vi "Fluence in multiple areas.vi"(0 "Analyze Fluence in":refnum<class "Analyze Fluence.lvclass">, 5 "Image in":T2, 7 "Energy":dbl[unit], 11 "error in (no error)":errorcluster) -> (4 "Analyze Fluence out":refnum<class "Analyze Fluence.lvclass">, 6 "Image Dst Out":T2, 8 "Max Fluence J/cm^2":dbl[unit], 10 "fluence infos":T3[](array[typedef]), 15 "error out":errorcluster)   [LabVIEW 2014, in "Analyze.lvlib" / "Analyze Fluence.lvclass"]
uses:
  Analyze Fluence.lvclass
  Fluence Info.ctl
  <vilib>/vision/Image Controls.llb/IMAQ Image.ctl
  Analyze Parameter/Analyze Parameter Fluence/Analyze Parameter Fluence.lvclass
  Analyze Fluence.lvclass/Analyze Fluence.ctl
  <vilib>/vision/NI_Vision_Development_Module.lvlib
  Analyze BaseClass/Analyze BaseClass/Analyze BaseClass.lvclass
panel:
  in  "ROI Descriptor out":T1 {"Contours"."Type" items=["No Selection", "Point", "Line", "Rectangle", "Oval", "Polygon", "Freehand Region", "Annulus", "Unused2", "Unused3", "Broken Line", "Freehand Line", "Rotated Rectangle"]}
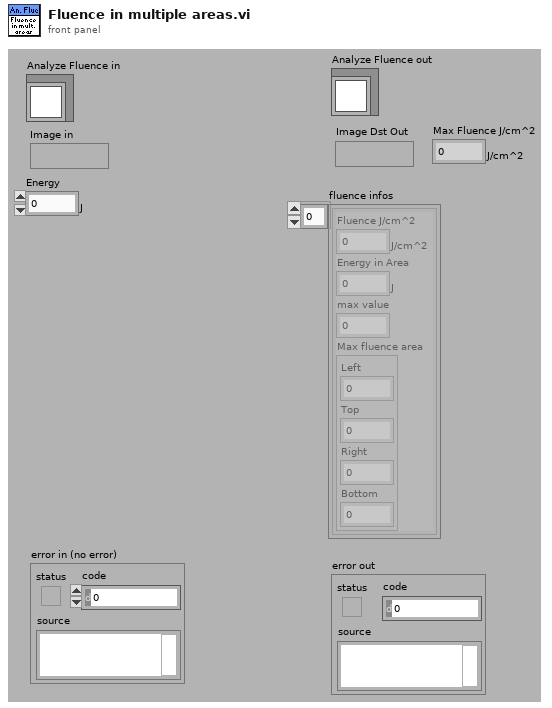
[diagram p1: front panel]
types:
  T1 = typedef "ROI Descriptor" = cluster{"Global Rectangle":i32[], "Contours":cluster{"ID":enum32{"External", "Internal"}, "Type":u32, "Coordinates":i32[]}[]}
  T2 = typedef "IMAQ Image.ctl" = refnum<image>
  T3 = typedef "Analyze.lvlib/Analyze Fluence.lvclass/Fluence Info.ctl" = cluster{"Fluence J/cm^2":dbl[unit], "Energy in Area":dbl[unit], "max value":i64, "Max fluence area":cluster{"Left":i32, "Top":i32, "Right":i32, "Bottom":i32}}
  T4 = typedef "Image Type" = u32
  T5 = typedef "IMAQ Rectangle" = cluster{"Left":i32, "Top":i32, "Right":i32, "Bottom":i32, "Rotation":dbl}
  T6 = cluster{"Left":i32, "Top":i32, "Right":i32, "Bottom":i32}
  T7 = cluster{"Fluence J/cm^2":dbl[unit], "Energy in Area":dbl[unit], "max value":i64, "Max fluence area":cluster{"Left":i32, "Top":i32, "Right":i32, "Bottom":i32}}
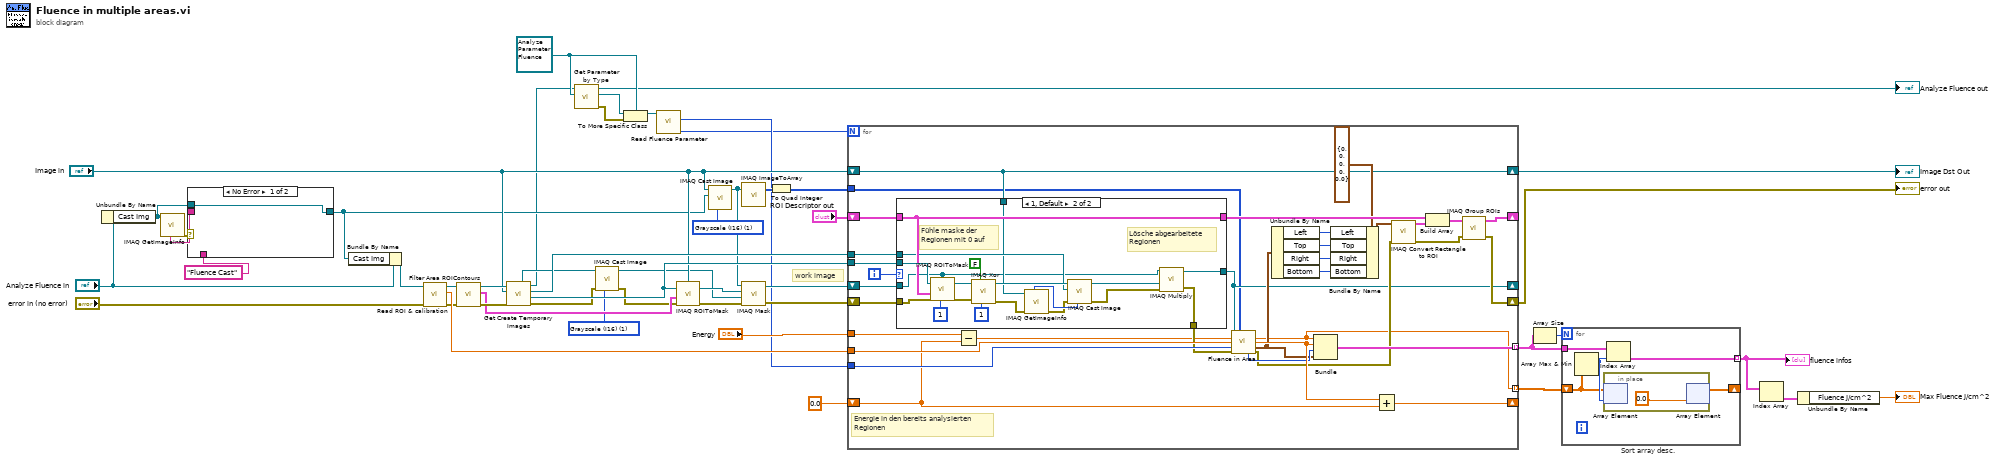
[diagram p0: block diagram]
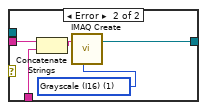
[diagram p3: hidden frame]
diagram:
  w5 = refnum<class "Analyze Parameter Fluence.lvclass"> refnum ("Parameter")
  w16 = T4 1 items=["Grayscale (U8)", "Grayscale (I16)", "Grayscale (SGL)", "Complex (CSG)", "RGB (U32)", "HSL (U32)", "RGB (U64)", "Grayscale (U16)"] ("Image Type")
  w26 = T4 1 items=["Grayscale (U8)", "Grayscale (I16)", "Grayscale (SGL)", "Complex (CSG)", "RGB (U32)", "HSL (U32)", "RGB (U64)", "Grayscale (U16)"] ("Image Type")
  # "work image"
  n1 = Unbundle By Name("Analyze Fluence in") -> ("Cast Img"=w21:T2)
  n2 = call "IMAQ GetImageInfo"("Image"=w21) -> ("error out"=w24:errorcluster, "Image Name"=w23:string)  [unwired: 3 in, 6 out]
  n3 = case shown="No Error" w24 {
    tunnel: w23 -> [_ w54]
    tunnel: "Fluence Cast" -> [_ w52]
    tunnel: [w50 w51] -> w19
    tunnel: w21 -> [w50 _]
    frame No Error {
    }
    frame Error {
      w55 = T4 1 items=["Grayscale (U8)", "Grayscale (I16)", "Grayscale (SGL)", "Complex (CSG)", "RGB (U32)", "HSL (U32)", "RGB (U64)", "Grayscale (U16)"] ("Image Type")
      n4 = Concatenate Strings(w54, w52) -> (w53:string)
      n5 = call "IMAQ Create"("Image Name"=w53, "Image Type"=w55) -> ("New Image"=w51:T2)  [unwired: 3 in, 1 out]
    }
  }
  n6 = Bundle By Name(cluster="Analyze Fluence in", "Cast Img"=w19) -> (w20:refnum<class "Analyze Fluence.lvclass">)
  n7 = call-dynamic "Read ROI & calibration.vi"("error in (no error)"="error in (no error)", "Analyze BaseClass in"=w20) -> ("error out"=w36:errorcluster, "calibration mm/px"=w40:dbl[unit], "Analyze BaseClass out"=w39:refnum<class "Analyze Fluence.lvclass">)  [unwired: 6 in, 1 out]
  n8 = call-dynamic "Filter Area ROIContours.vi"("error in (no error)"=w36, "Analyze BaseClass in"=w39) -> ("error out"=w35:errorcluster, "ROI of Area type"=w29:T1, "Analyze BaseClass out"=w38:refnum<class "Analyze Fluence.lvclass">)  [unwired: 7 in]
  n9 = call-dynamic "Get Create Temporary Images.vi"("error in (no error)"=w35, "Image in"="Image in", "Analyze BaseClass in"=w38) -> ("error out"=w15:errorcluster, "image mask"=w41:T2, "work image"=w32:T2, "Analyze BaseClass out"=w3:refnum<class "Analyze Fluence.lvclass">, "masked image"=w18:T2)  [unwired: 4 in]
  n10 = call "Get Parameter by Type.vi"("Parameter Type"=w5, "Analyze BaseClass in"=w3) -> ("error out"=w6:errorcluster, "Parameter"=w4:refnum<class "Analyze Parameter Base.lvclass">, "Analyze BaseClass out"=→"Analyze Fluence out":refnum<class "Analyze Fluence.lvclass">)  [unwired: 6 in, 1 out]
  n11 = call "IMAQ Cast Image"("Image Type"=w16, "error in (no error)"=w15, "Image Src"=w18) -> ("error out"=w14:errorcluster, "Image Dst Out"=w17:T2)  [unwired: 7 in]
  n12 = To More Specific Class(target class=w5, reference=w4, error in=w6) -> (specific class reference=w1:refnum<class "Analyze Parameter Fluence.lvclass">)  [unwired: 1 out]
  n13 = call "Read Fluence Parameter.vi"("Analyze Parameter Fluence in"=w1) -> ("#of Areas"=w7:i32, "Size of region (px)"=w8:i32)  [unwired: 7 in, 2 out]
  n14 = call "IMAQ ROIToMask"("error in (no error)"=w14, "ROI Descriptor"=w29, "Image"=w41, "Image Model"="Image in") -> ("error out"=w42:errorcluster, "Image Out"=w48:T2)  [unwired: 2 in, 1 out]
  n15 = call "IMAQ Cast Image"("Image Type"=w26, "Image Dst"=w19, "Image Src"="Image in") -> ("Image Dst Out"=w27:T2)  [unwired: 7 in, 1 out]
  n16 = call "IMAQ ImageToArray"("Image"=w27) -> ("Image Pixels (I16)"=w31:i16[][])  [unwired: 3 in, 4 out]
  n17 = call "IMAQ Mask"("error in (no error)"=w42, "Image Dst"=w17, "Image Mask"=w48, "Image Src"=w27) -> ("error out"=w33:errorcluster, "Image Dst Out"=w34:T2)  [unwired: 1 in]
  n18 = To Quad Integer(1:w31) -> (0:w30:i64[][])
  n19 = for {
    N: w7 -> [_]
    tunnel: "Energy" -> [w89]
    tunnel: w40 -> [w88]
    tunnel: w8 -> [w87]
    shift-right: [w86] -> _
    shift-left: "ROI Descriptor out" -> [w80]
    tunnel: w41 -> [w85]
    tunnel: w32 -> [w83]
    shift-right: [w59] -> _
    shift-left: w34 -> [w60]
    shift-right: [w63] -> w43
    shift-left: w33 -> [w84]
    shift-right: [w82] -> _
    shift-left: dbl[unit] 0.0 ("Energy in Area") -> [w81]
    tunnel: [w61] -> w10 mode=indexing
    shift-right: [w57] -> w44
    shift-left: "Image in" -> [w57]
    tunnel: [w64] -> w11 mode=indexing
    tunnel: w30 -> [w56]
    i -> [w67]
    # "Energie in den bereits analysierten \nRegionen"
    n20 = case shown="1, Default" w67 {
      tunnel: w85 -> [_ w107]
      tunnel: w84 -> [w92 w106]
      tunnel: w83 -> [_ w95]
      tunnel: w60 -> [w91 w93]
      tunnel: w80 -> [w90 w99]
      tunnel: [w92 w109] -> w72
      tunnel: [w91 w108] -> w59
      tunnel: [w90 w99] -> w65
      tunnel: w57 -> [_ w94]
      frame 0 {
      }
      frame 1, Default {
        # "Lösche abgearbeitete\nRegionen"
        # "Fühle maske der\nRegionen mit 0 auf"
        n21 = call "IMAQ ROIToMask"("error in (no error)"=w106, "ROI Descriptor"=w99, "Filling Value (255)"=1 ("Background Value (0)"), "Image"=w107, "Image Model"=w93) -> ("error out"=w102:errorcluster, "Image Out"=w101:T2)  [unwired: 1 in, 1 out]
        n22 = call "IMAQ Xor"("Constant"=1, "Xor/Xnor (Xor)"=FALSE ("And/Nand (And)"), "error in (no error)"=w102, "Image Src A"=w101) -> ("error out"=w97:errorcluster, "Image Dst Out"=w100:T2)  [unwired: 6 in]
        n23 = call "IMAQ GetImageInfo"("error in (no error)"=w97, "Image"=w94) -> ("error out"=w96:errorcluster, "Image Type"=w98:T4)  [unwired: 2 in, 6 out]
        n24 = call "IMAQ Cast Image"("Image Type"=w98, "error in (no error)"=w96, "Image Dst"=w95, "Image Src"=w100) -> ("error out"=w110:errorcluster, "Image Dst Out"=w111:T2)  [unwired: 6 in]
        n25 = call "IMAQ Multiply"("Image Src A"=w93, "Image Src B"=w111, "error in (no error)"=w110) -> ("Image Dst Out"=w108:T2, "error out"=w109:errorcluster)  [unwired: 4 in]
      }
    }
    n26 = Subtract(x=w89, y=w81) -> (x-y=w71:dbl[unit])
    n27 = call "Fluence in Area.vi"("Masked Image (I16only)"=w59, "Origin Image"=w56, "Energie"=w71, "calibration mm/px"=w88, "Size of region"=w87, "error in (no error)"=w72) -> ("Fluence J/cm^2"=w61:dbl[unit], "Energy in Area"=w70:dbl[unit], "Max fluence area"=w68:T6, "max value"=w69:i64, "error out"=w62:errorcluster)  [unwired: 5 in]
    n28 = Unbundle By Name(w68) -> ("Left"=w76:i32, "Top"=w77:i32, "Right"=w78:i32, "Bottom"=w79:i32)
    n29 = Bundle("Fluence J/cm^2"=w61, "Energy in Area"=w70, "max value"=w69, "Max fluence area"=w68) -> (w64:T7)  [unwired: 1 in]
    n30 = Bundle By Name(cluster=T5 {"Left"=0, "Top"=0, "Right"=0, "Bottom"=0, "Rotation"=0.0} ("Rectangle"), "Left"=w76, "Top"=w77, "Right"=w78, "Bottom"=w79) -> (w75:T5)
    n31 = Add(x=w70, y=w81) -> (x+y=w82:dbl[unit])
    n32 = call "IMAQ Convert Rectangle to ROI"("error in (no error)"=w62, "Rectangle"=w75) -> ("error out"=w66:errorcluster, "ROI Descriptor"=w74:T1)  [unwired: 7 in]
    n33 = Build Array(w65, w74) -> (w73:T1[])
    n34 = call "IMAQ Group ROIs"("error in (no error)"=w66, "ROI Descriptors"=w73) -> ("error out"=w63:errorcluster, "ROI Descriptor out"=w86:T1)  [unwired: 2 in]
  }
  "error out" <- w43
  "Image Dst Out" <- w44
  n35 = Array Size(array=w11) -> (size(s)=w12:i32)
  n36 = for "Sort array desc." {
    N: w12 -> [_]
    shift-right: [w112] -> _
    shift-left: w10 -> [w113]
    tunnel: w11 -> [w116]
    tunnel: [w115] -> w45 mode=indexing
    n37 = Array Max & Min(array=w113) -> (max index (indices)=w114:i32)  [unwired: 3 out]
    n38 = in-place {
      n39 = in-place-array #1(w113, w114) -> ()  [unwired: 1 out]
      n40 = in-place-array #1(dbl[unit] 0.0 ("element")) -> (w112:dbl[unit][])  [unwired: 1 out]
    }
    n41 = Index Array(array=w116, index=w114) -> (element=w115:T7)
  }
  "fluence infos" <- w45
  n42 = Index Array(array=w45) -> (element=w47:T7)  [unwired: 1 in]
  n43 = Unbundle By Name(w47) -> ("Fluence J/cm^2"=→"Max Fluence J/cm^2":dbl[unit])
